vi "多参数据转列表.vi"(7 "参数名":string, 11 "测量数据块":T1) -> (3 "添加的数组":string[][](array[string]))   [LabVIEW 2016, in "斯坦道原位多参数.lvlib"]
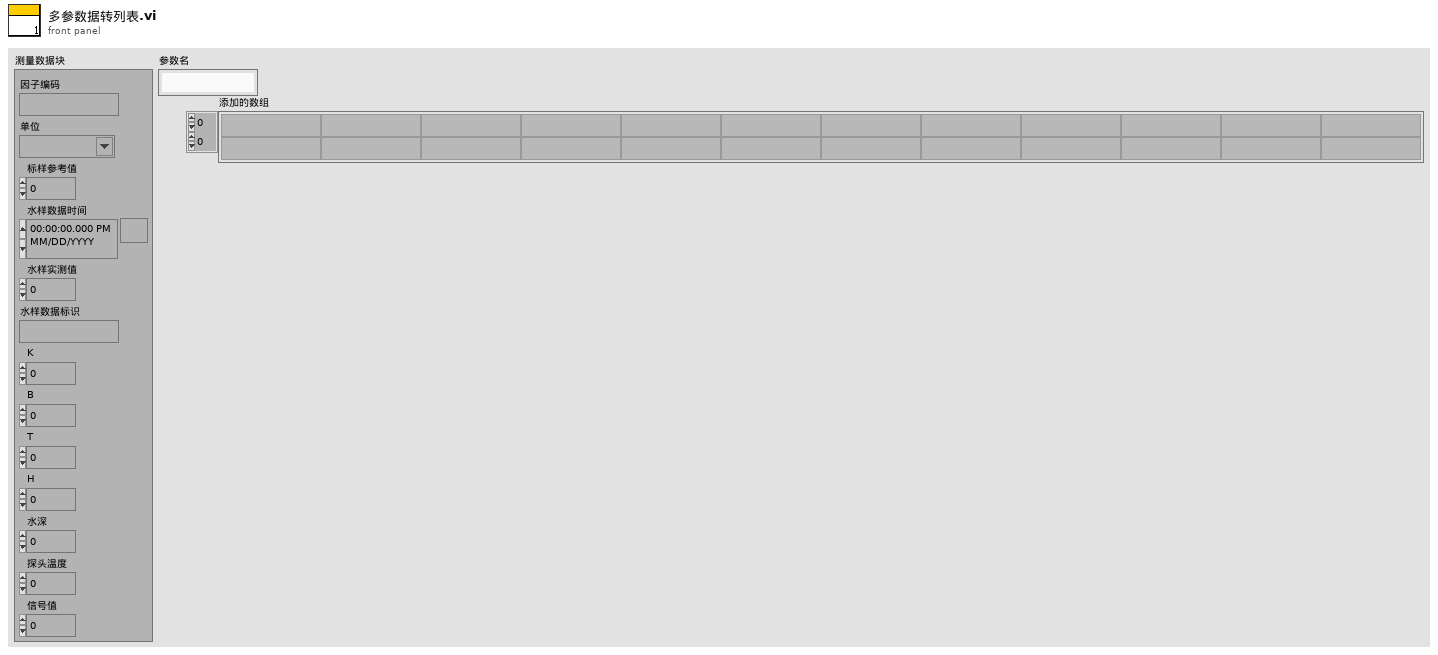
[diagram p1: front panel]
types:
  T1 = cluster{"因子编码":string, "单位":string, "标样参考值":sgl, "水样数据时间":timestamp, "水样实测值":sgl, "水样数据标识":string, "K":sgl, "B":sgl, "T":sgl, "H":sgl, "水深":sgl, "探头温度":sgl, "信号值":sgl}
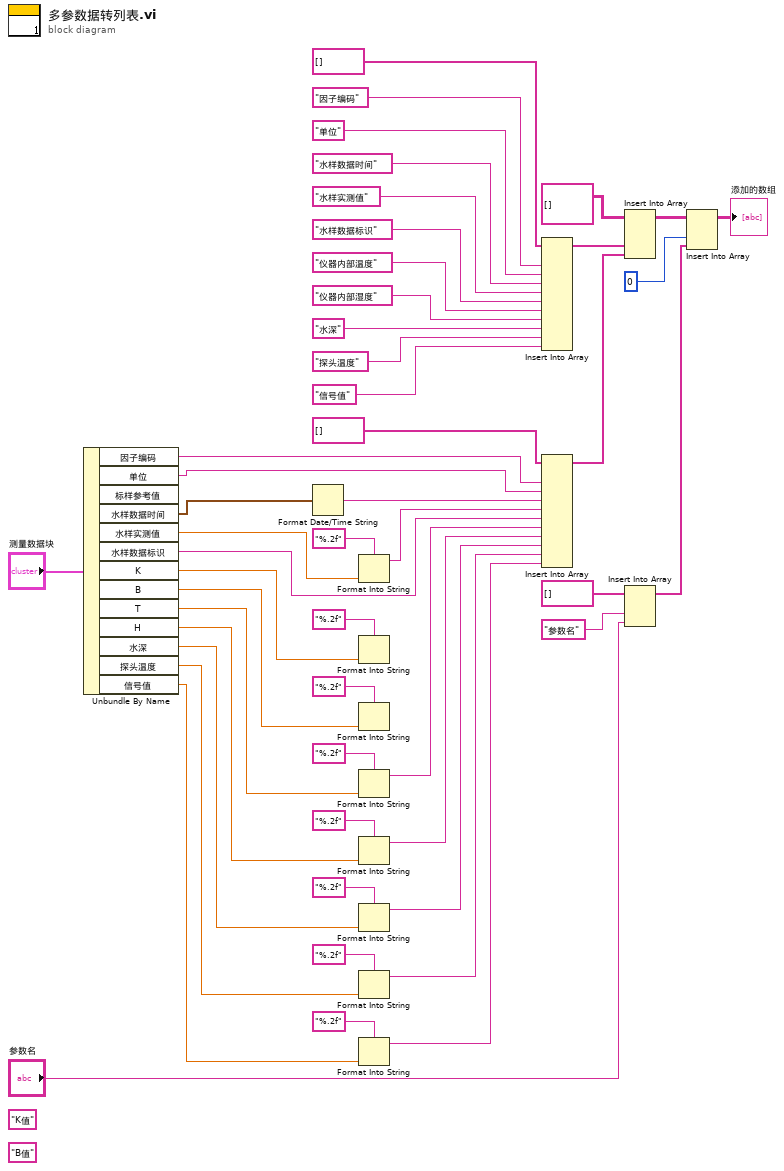
[diagram p0: block diagram]
diagram:
  (unwired) "B值"
  (unwired) "K值"
  n1 = Unbundle By Name("测量数据块") -> ("因子编码"=w36:string, "单位"=w35:string, "水样数据时间"=w34:timestamp, "水样实测值"=w33:sgl, "水样数据标识"=w32:string, "K"=w26:sgl, "B"=w25:sgl, "T"=w24:sgl, "H"=w23:sgl, "水深"=w22:sgl, "探头温度"=w13:sgl, "信号值"=w2:sgl)  [unwired: 1 out]
  n2 = Format Date/Time String(seconds (now)=w34) -> (date/time string=w48:string)  [unwired: 2 in]
  n3 = Format Into String(format string="%.2f" ("格式字符串"), w33) -> (resulting string=w47:string)  [unwired: 2 in, 1 out]
  n4 = Format Into String(format string="%.2f" ("格式字符串"), w26) -> ()  [unwired: 2 in, 2 out]
  n5 = Format Into String(format string="%.2f" ("格式字符串"), w25) -> ()  [unwired: 2 in, 2 out]
  n6 = Format Into String(format string="%.2f" ("格式字符串"), w24) -> (resulting string=w8:string)  [unwired: 2 in, 1 out]
  n7 = Format Into String(format string="%.2f" ("格式字符串"), w23) -> (resulting string=w7:string)  [unwired: 2 in, 1 out]
  n8 = Format Into String(format string="%.2f" ("格式字符串"), w22) -> (resulting string=w6:string)  [unwired: 2 in, 1 out]
  n9 = Format Into String(format string="%.2f" ("格式字符串"), w13) -> (resulting string=w5:string)  [unwired: 2 in, 1 out]
  n10 = Format Into String(format string="%.2f" ("格式字符串"), w2) -> (resulting string=w1:string)  [unwired: 2 in, 1 out]
  n11 = Insert Into Array(array=string[] [], new element #1="因子编码", new element #2="单位", new element #3="水样数据时间", new element #4="水样实测值", new element #5="水样数据标识", new element #6="仪器内部温度", new element #7="仪器内部湿度", new element #8="水深", new element #9="探头温度", new element #10="信号值") -> (w39:string[])  [unwired: 1 in]
  n12 = Insert Into Array(array=string[] [] ("数组"), new element #1=w36, new element #2=w35, new element #3=w48, new element #4=w47, new element #5=w32, new element #6=w8, new element #7=w7, new element #8=w6, new element #9=w5, new element #10=w1) -> (w38:string[])  [unwired: 1 in]
  n13 = Insert Into Array(array=string[][] [], new element #1=w39, new element #2=w38) -> (w21:string[][])  [unwired: 2 in]
  n14 = Insert Into Array(array=string[] [] ("新元素/子数组"), new element #1="参数名" ("新元素/子数组"), new element #2="参数名") -> (w17:string[])  [unwired: 1 in]
  n15 = Insert Into Array(array=w21, index (col)=0 ("禁用的索引 (列)"), new element=w17) -> (→"添加的数组":string[][])  [unwired: 1 in]
